vi "Variant Tree Test VI.vi"() -> ()   [LabVIEW 2017]
uses:
  Variant Tree.xctl
panel:
  in  "Cluster":T1
  out "Variant":variant
  in  "stop":bool
  in  "Variant Tree":variant(xcontrol)
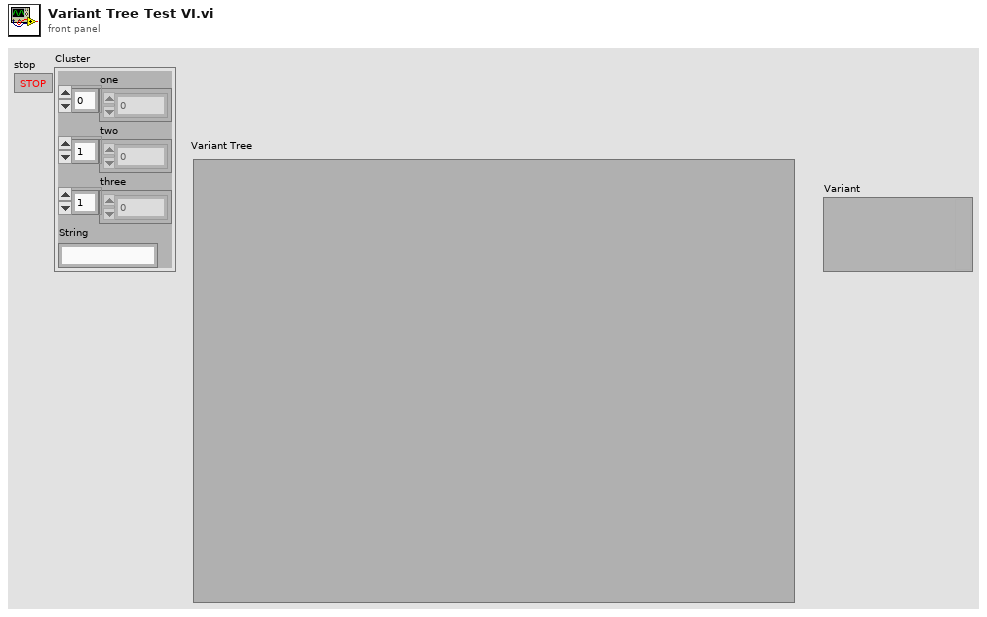
[diagram p1: front panel]
types:
  T1 = cluster{"one":u16[], "two":i32[], "three":u8[], "String":string}
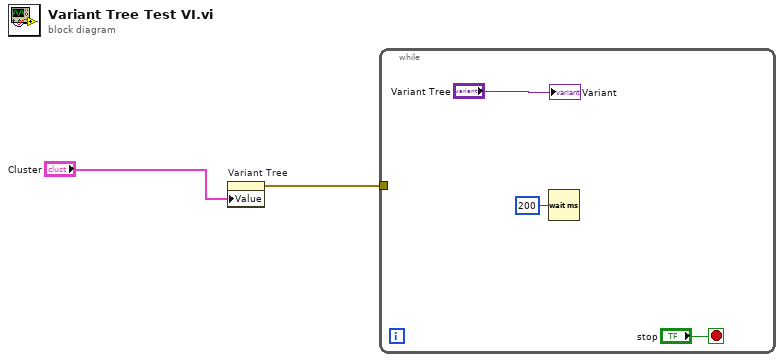
[diagram p0: block diagram]
diagram:
  n1 = property on="Variant Tree" class="Variant Tree (strict)"("Value"="Cluster") -> (error out=w2:errorcluster)  [unwired: 2 in, 1 out]
  n2 = while {
    tunnel: w2 -> [_]
    stop <- "stop" stop-if-true
    n3 = Wait (ms)(milliseconds to wait=u32 200) -> ()  [unwired: 1 out]
    "Variant" <- "Variant Tree"
  }
